vi "TAT-Main.vi"() -> ()   [LabVIEW 2017]
panel:
  in  "Modify SN":bool
  in  "PRINT":bool
  in  "Torque IO Status":bool
  in  "Ass IO Status":bool
  in  "Recipe":bool
  out "error out":errorcluster
  in  "Logout":bool
  in  "Stop":bool
  in  "Create Login":bool
  in  "Reports":bool
  in  "Start":bool
  out "Time":string
  out "Date":string
  in  "Login":bool
  # "RBC ORVM- TRACEABILITY, SCANNING & BARCODE PRINTING"
  # "KAPSE SONS ROBOTICS\n& AUTOMATION"
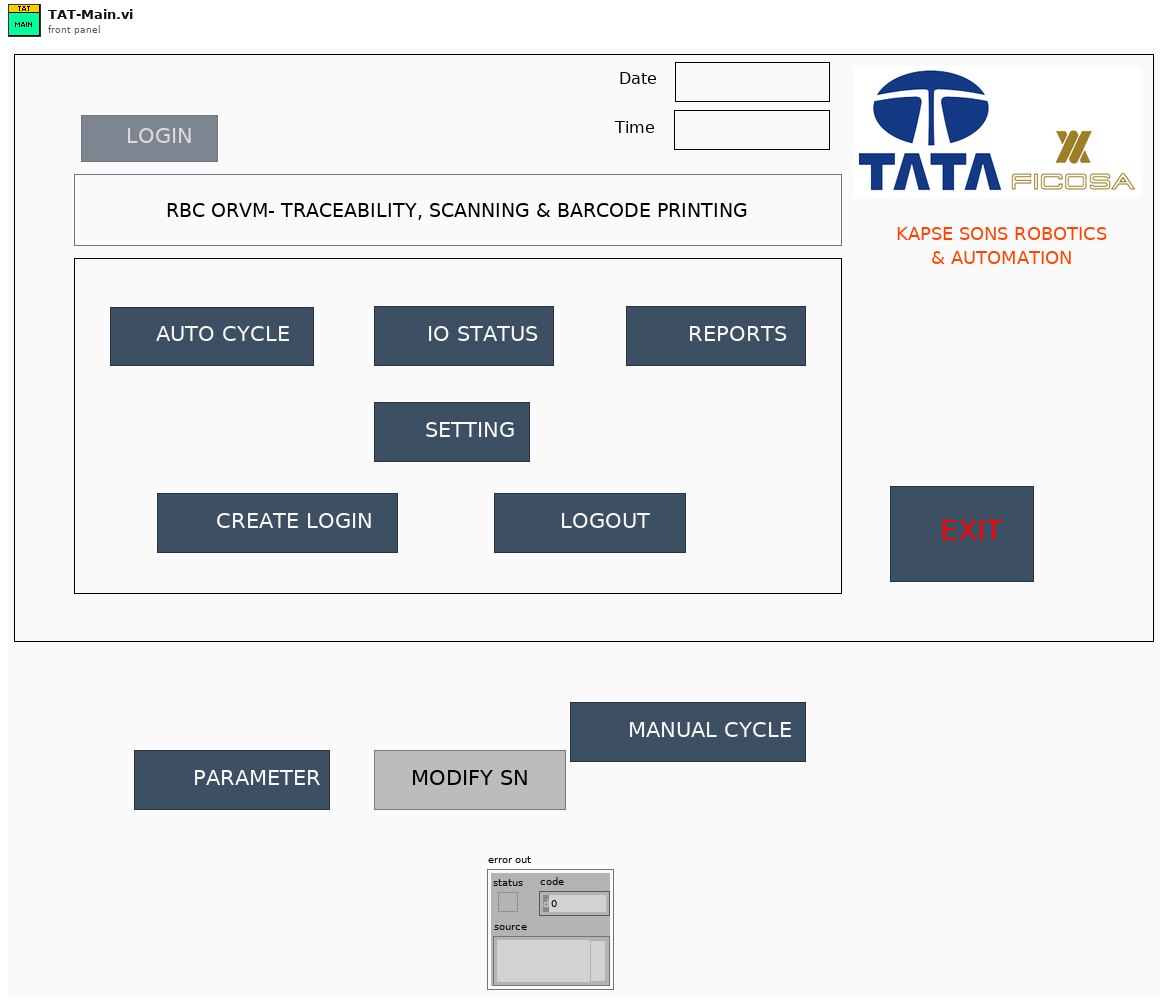
[diagram p1: front panel]
types:
  T1 = enum8{"Enabled", "Disabled", "Disabled and Grayed Out"}
  T2 = enum32{"Invalid", "Standard", "Closed", "Hidden", "Minimized", "Maximized"}
  T3 = enum32{"invalid app kind", "Development System", "Run Time System", "Student Edition", "Embedded LabVIEW", "Evaluation", "Custom"}
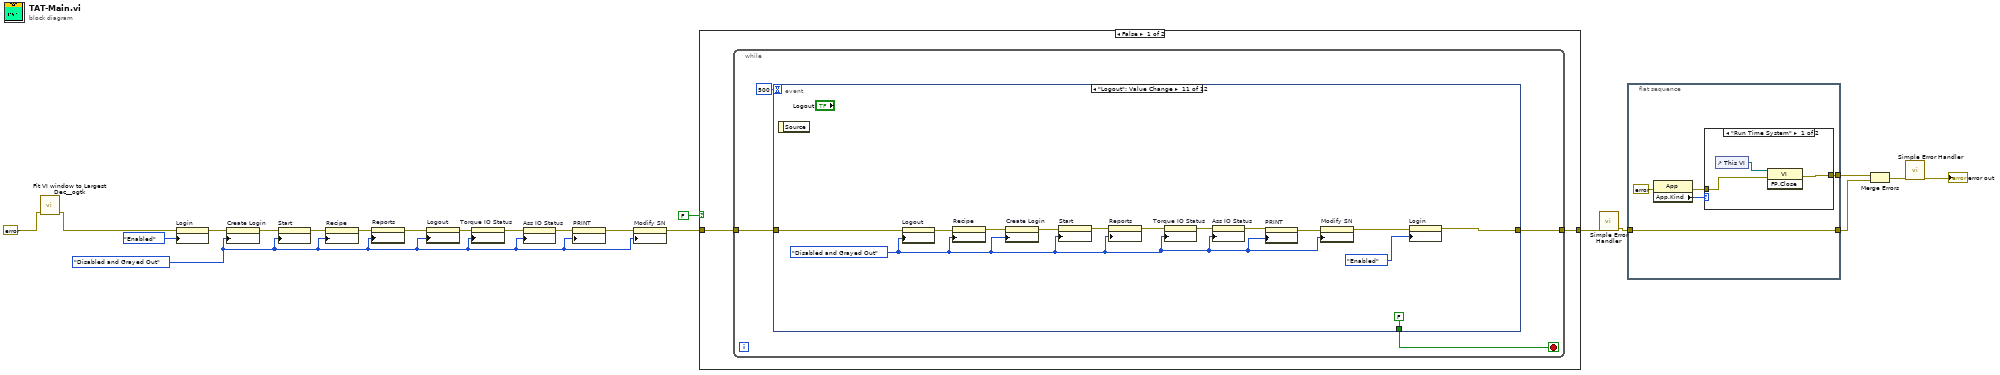
[diagram p0: block diagram]
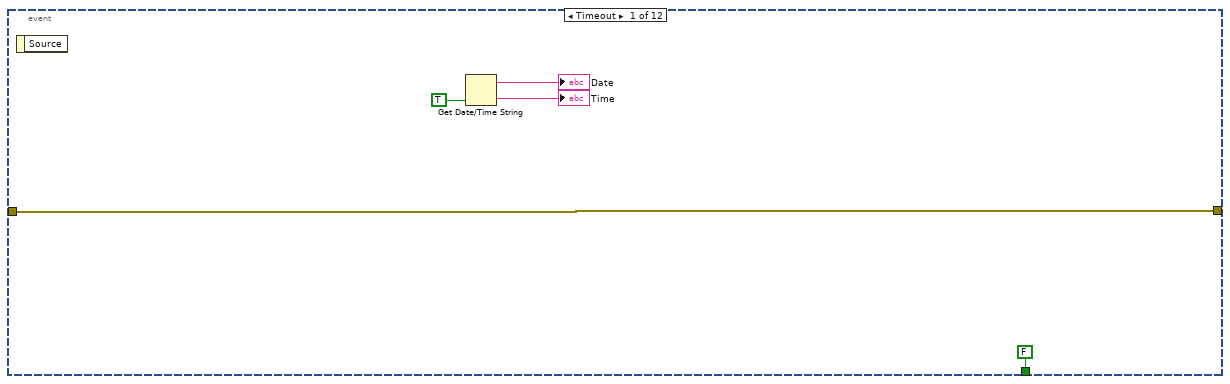
[diagram p3: hidden frame]
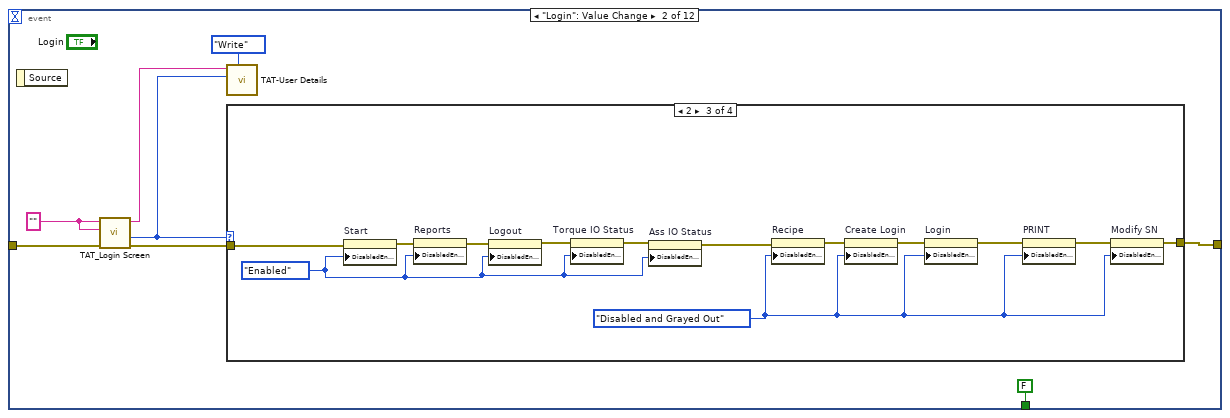
[diagram p4: hidden frame]
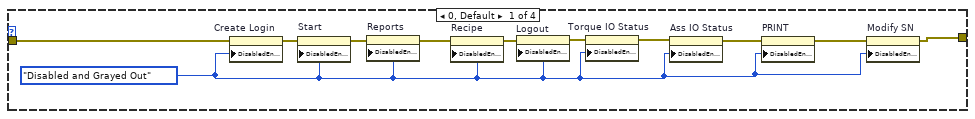
[diagram p5: hidden frame]
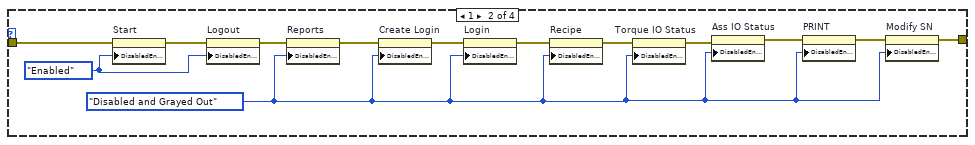
[diagram p6: hidden frame]
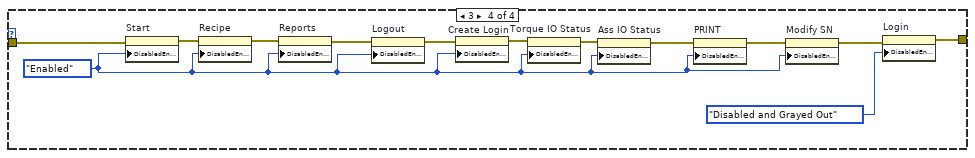
[diagram p7: hidden frame]
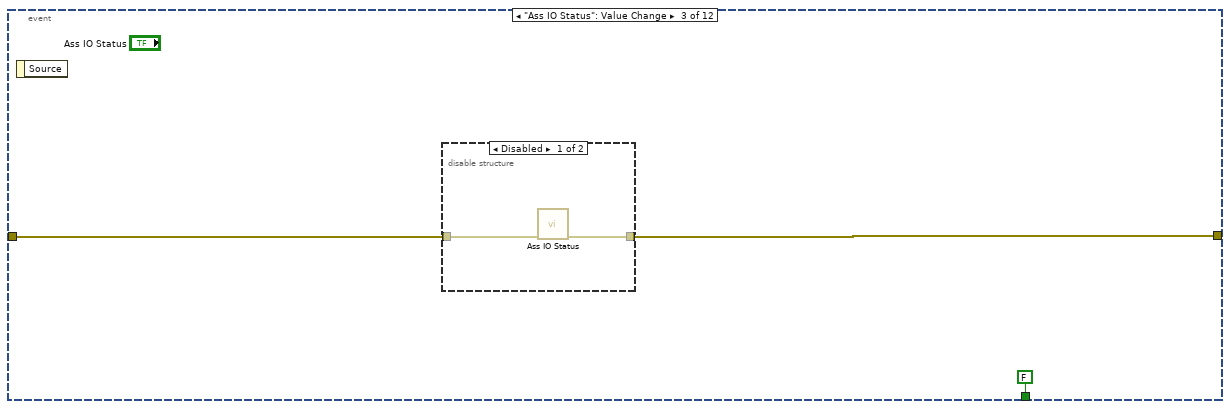
[diagram p8: hidden frame]
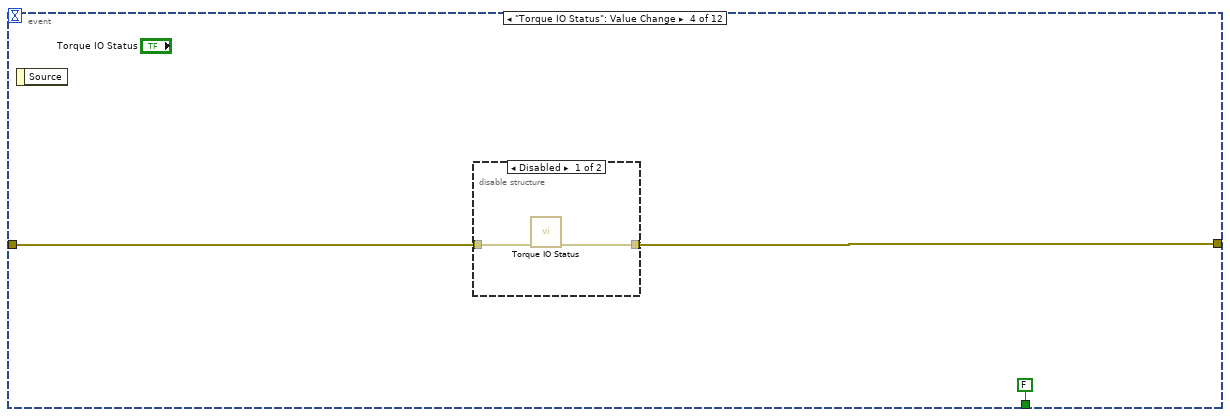
[diagram p10: hidden frame]
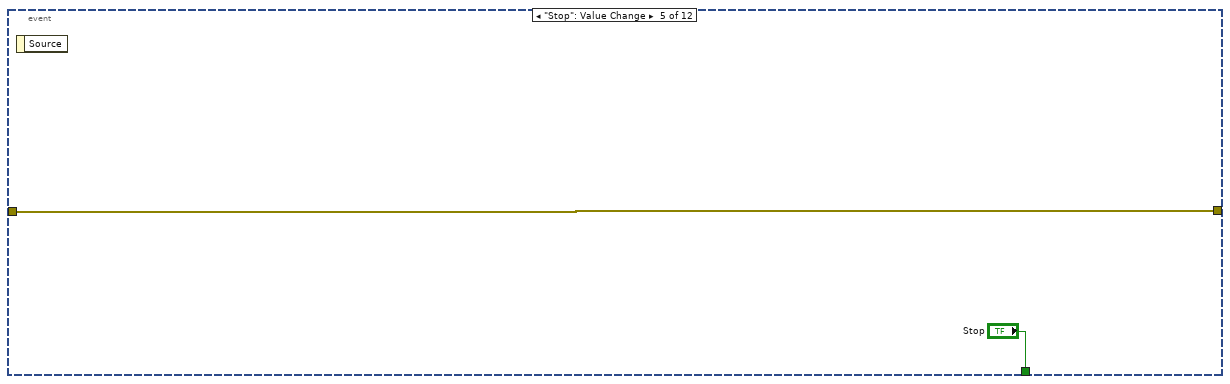
[diagram p12: hidden frame]
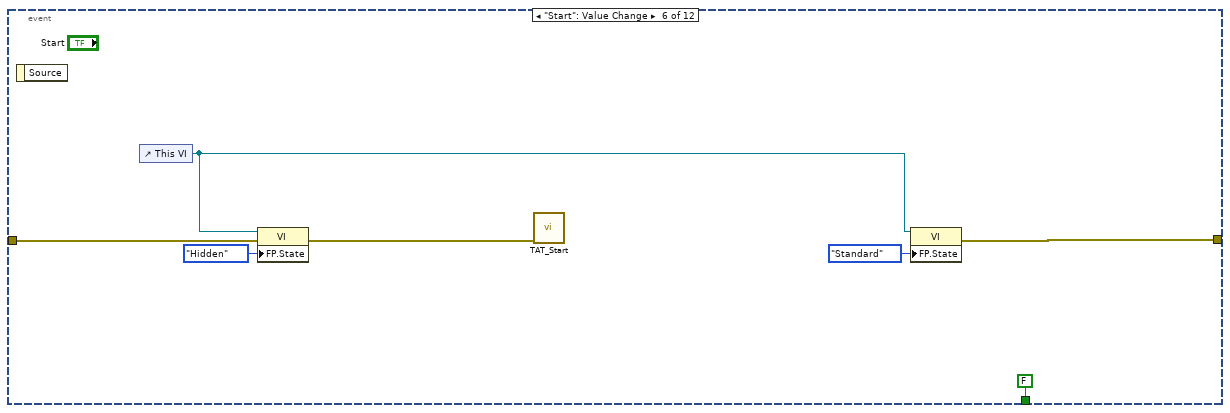
[diagram p13: hidden frame]
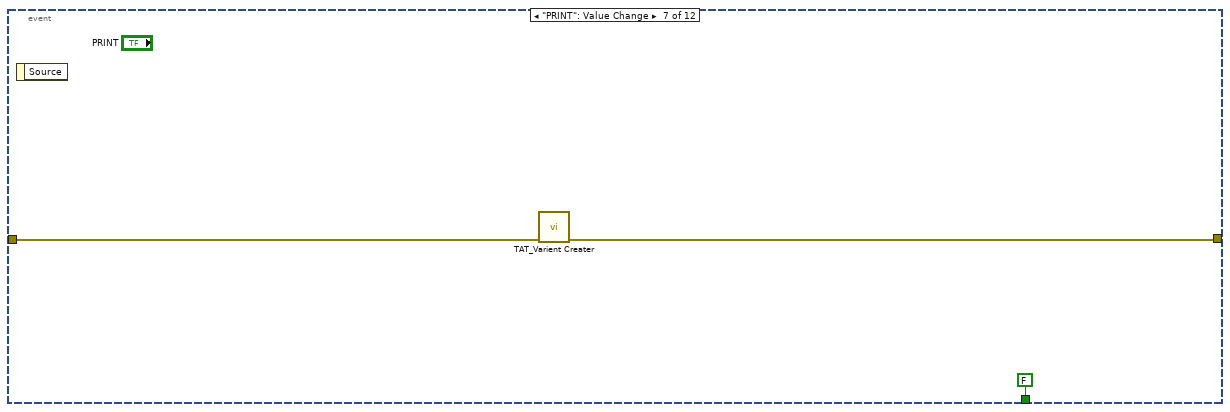
[diagram p14: hidden frame]
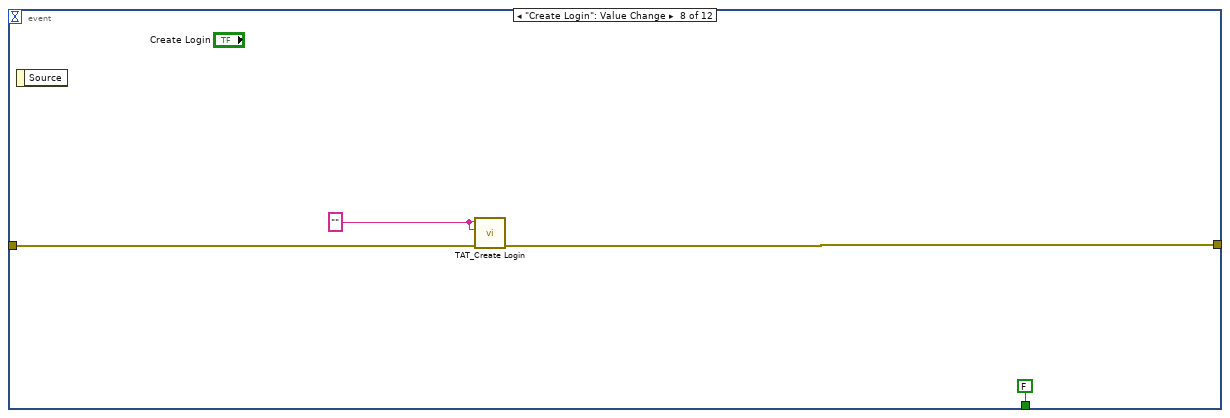
[diagram p15: hidden frame]
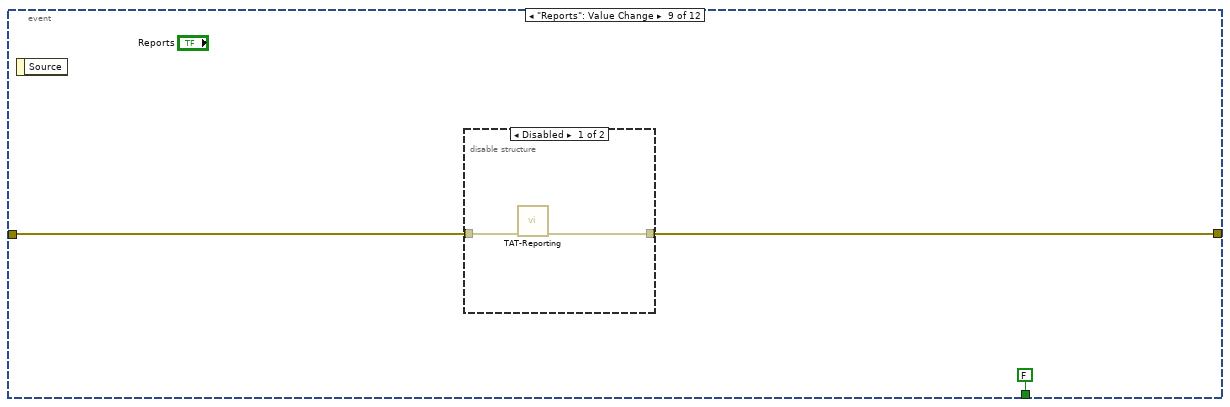
[diagram p16: hidden frame]
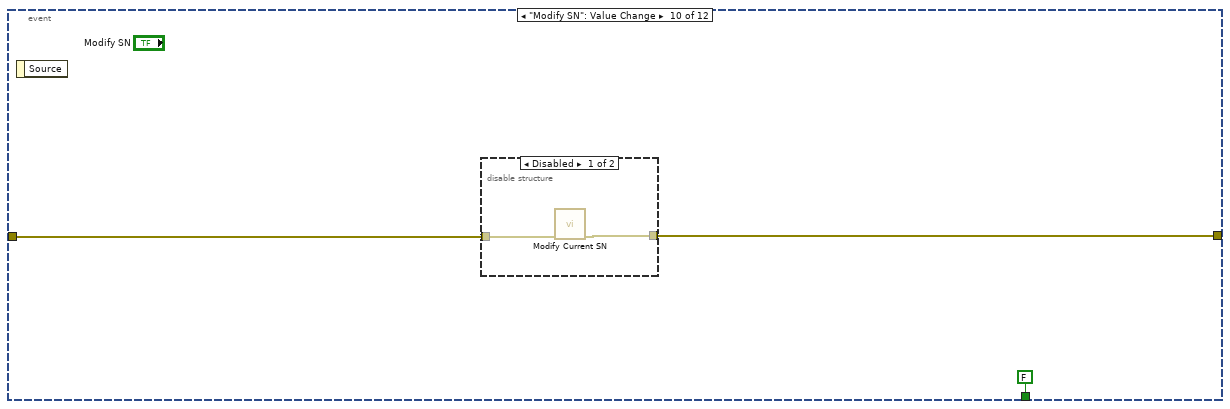
[diagram p18: hidden frame]
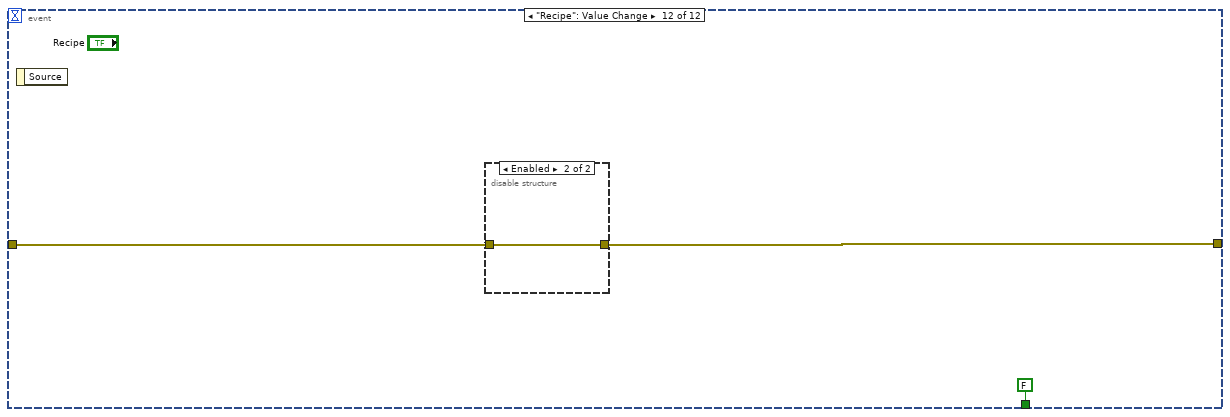
[diagram p20: hidden frame]
diagram:
  w4 = T1."Disabled and Grayed Out" ("Disabled")
  n1 = call <userlib>:"Fit VI window to Largest Dec__ogtk.vi"("error in (no error)"=errorcluster {"status"=FALSE, "code"=0, "source"=""} ("error constant")) -> ("error out"=w1:errorcluster)  [unwired: 5 in, 1 out]
  n2 = property on="Login" class="Bool"(error in=w1, "DisabledEnum"=T1."Enabled" ("Disabled")) -> (error out=w15:errorcluster)  [unwired: 1 in, 1 out]
  n3 = property on="Create Login" class="Bool"(error in=w15, "DisabledEnum"=w4) -> (error out=w20:errorcluster)  [unwired: 1 in, 1 out]
  n4 = property on="Start" class="Bool"(error in=w20, "DisabledEnum"=w4) -> (error out=w11:errorcluster)  [unwired: 1 in, 1 out]
  n5 = property on="Recipe" class="Bool"(error in=w11, "DisabledEnum"=w4) -> (error out=w10:errorcluster)  [unwired: 1 in, 1 out]
  n6 = property on="Reports" class="Bool"(error in=w10, "DisabledEnum"=w4) -> (error out=w13:errorcluster)  [unwired: 1 in, 1 out]
  n7 = property on="Logout" class="Bool"(error in=w13, "DisabledEnum"=w4) -> (error out=w9:errorcluster)  [unwired: 1 in, 1 out]
  n8 = property on="Torque IO Status" class="Bool"(error in=w9, "DisabledEnum"=w4) -> (error out=w8:errorcluster)  [unwired: 1 in, 1 out]
  n9 = property on="Ass IO Status" class="Bool"(error in=w8, "DisabledEnum"=w4) -> (error out=w7:errorcluster)  [unwired: 1 in, 1 out]
  n10 = property on="PRINT" class="Bool"(error in=w7, "DisabledEnum"=w4) -> (error out=w6:errorcluster)  [unwired: 1 in, 1 out]
  n11 = property on="Modify SN" class="Bool"(error in=w6, "DisabledEnum"=w4) -> (error out=w5:errorcluster)  [unwired: 1 in, 1 out]
  n12 = case shown="False" FALSE {
    tunnel: w5 -> [w23 w147]
    tunnel: [w22 w147] -> w21
    frame False {
      n13 = while {
        tunnel: w23 -> [w26]
        tunnel: [w25] -> w22
        stop <- w24 stop-if-true
        n14 = event shown="[10] \"Logout\": Value Change" {
          selector: _ -> [_ _ _ _ _ _ _ _ _ _ _ _]
          dyn-events: _ -> [_ _ _ _ _ _ _ _ _ _ _ _]
          timeout: 500 -> [_ _ _ _ _ _ _ _ _ _ _ _]
          tunnel: w26 -> [w30 w40 w93 w97 w101 w107 w111 w116 w119 w124 w137 w143]
          tunnel: [w30 w38 w92 w96 w101 w104 w110 w115 w118 w123 w138 w142] -> w25
          tunnel: [FALSE ("Stop") FALSE ("Stop") FALSE ("Stop") FALSE ("Stop") "Stop" FALSE ("Stop") FALSE ("Stop") FALSE ("Stop") FALSE ("Stop") FALSE ("Stop") FALSE ("Stop") FALSE ("Stop")] -> w24
          event Timeout {
            n15 = event-data() -> ()  [unwired: 1 in, 1 out]
            n16 = Get Date/Time String(want seconds? (F)=TRUE) -> (date string=→"Date":string, time string=→"Time":string)  [unwired: 2 in]
          }
          event "Login": Value Change {
            w35 = "" ("User Name")
            n17 = event-data() -> ()  [unwired: 1 in, 1 out]
            n18 = call "TAT_Login Screen.vi"("Error In"=w40, "Password"=w35, "User Name"=w35) -> ("error out"=w39:errorcluster, "Level"=w33:i32, "User Name Out"=w36:string)  [unwired: 5 in, 1 out]
            n19 = call "TAT-User Details.vi"("Enum"=enum16{"Read", "Write"}."Write", "Level In"=w33, "User Name In"=w36) -> ()  [unwired: 7 in, 2 out]
            n20 = case shown="2" w33 {
              tunnel: w39 -> [w49 w64 w77 w90]
              tunnel: [w42 w53 w66 w89] -> w38
              frame 0, Default {
                w41 = T1."Disabled and Grayed Out" ("Disabled")
                n21 = property on="Create Login" class="Bool"(error in=w49, "DisabledEnum"=w41) -> (error out=w51:errorcluster)  [unwired: 1 in, 1 out]
                n22 = property on="Start" class="Bool"(error in=w51, "DisabledEnum"=w41) -> (error out=w50:errorcluster)  [unwired: 1 in, 1 out]
                n23 = property on="Reports" class="Bool"(error in=w50, "DisabledEnum"=w41) -> (error out=w48:errorcluster)  [unwired: 1 in, 1 out]
                n24 = property on="Recipe" class="Bool"(error in=w48, "DisabledEnum"=w41) -> (error out=w47:errorcluster)  [unwired: 1 in, 1 out]
                n25 = property on="Logout" class="Bool"(error in=w47, "DisabledEnum"=w41) -> (error out=w46:errorcluster)  [unwired: 1 in, 1 out]
                n26 = property on="Torque IO Status" class="Bool"(error in=w46, "DisabledEnum"=w41) -> (error out=w45:errorcluster)  [unwired: 1 in, 1 out]
                n27 = property on="Ass IO Status" class="Bool"(error in=w45, "DisabledEnum"=w41) -> (error out=w44:errorcluster)  [unwired: 1 in, 1 out]
                n28 = property on="PRINT" class="Bool"(error in=w44, "DisabledEnum"=w41) -> (error out=w43:errorcluster)  [unwired: 1 in, 1 out]
                n29 = property on="Modify SN" class="Bool"(error in=w43, "DisabledEnum"=w41) -> (error out=w42:errorcluster)  [unwired: 1 in, 1 out]
              }
              frame 1 {
                w52 = T1."Disabled and Grayed Out" ("Disabled")
                w60 = T1."Enabled" ("Disabled")
                n30 = property on="Start" class="Bool"(error in=w64, "DisabledEnum"=w60) -> (error out=w59:errorcluster)  [unwired: 1 in, 1 out]
                n31 = property on="Logout" class="Bool"(error in=w59, "DisabledEnum"=w60) -> (error out=w62:errorcluster)  [unwired: 1 in, 1 out]
                n32 = property on="Reports" class="Bool"(error in=w62, "DisabledEnum"=w52) -> (error out=w63:errorcluster)  [unwired: 1 in, 1 out]
                n33 = property on="Create Login" class="Bool"(error in=w63, "DisabledEnum"=w52) -> (error out=w61:errorcluster)  [unwired: 1 in, 1 out]
                n34 = property on="Login" class="Bool"(error in=w61, "DisabledEnum"=w52) -> (error out=w58:errorcluster)  [unwired: 1 in, 1 out]
                n35 = property on="Recipe" class="Bool"(error in=w58, "DisabledEnum"=w52) -> (error out=w56:errorcluster)  [unwired: 1 in, 1 out]
                n36 = property on="Torque IO Status" class="Bool"(error in=w56, "DisabledEnum"=w52) -> (error out=w57:errorcluster)  [unwired: 1 in, 1 out]
                n37 = property on="Ass IO Status" class="Bool"(error in=w57, "DisabledEnum"=w52) -> (error out=w55:errorcluster)  [unwired: 1 in, 1 out]
                n38 = property on="PRINT" class="Bool"(error in=w55, "DisabledEnum"=w52) -> (error out=w54:errorcluster)  [unwired: 1 in, 1 out]
                n39 = property on="Modify SN" class="Bool"(error in=w54, "DisabledEnum"=w52) -> (error out=w53:errorcluster)  [unwired: 1 in, 1 out]
              }
              frame 2 {
                w65 = T1."Disabled and Grayed Out" ("Disabled")
                w69 = T1."Enabled" ("Disabled")
                n40 = property on="Start" class="Bool"(error in=w77, "DisabledEnum"=w69) -> (error out=w74:errorcluster)  [unwired: 1 in, 1 out]
                n41 = property on="Reports" class="Bool"(error in=w74, "DisabledEnum"=w69) -> (error out=w76:errorcluster)  [unwired: 1 in, 1 out]
                n42 = property on="Logout" class="Bool"(error in=w76, "DisabledEnum"=w69) -> (error out=w71:errorcluster)  [unwired: 1 in, 1 out]
                n43 = property on="Torque IO Status" class="Bool"(error in=w71, "DisabledEnum"=w69) -> (error out=w72:errorcluster)  [unwired: 1 in, 1 out]
                n44 = property on="Ass IO Status" class="Bool"(error in=w72, "DisabledEnum"=w69) -> (error out=w70:errorcluster)  [unwired: 1 in, 1 out]
                n45 = property on="Recipe" class="Bool"(error in=w70, "DisabledEnum"=w65) -> (error out=w73:errorcluster)  [unwired: 1 in, 1 out]
                n46 = property on="Create Login" class="Bool"(error in=w73, "DisabledEnum"=w65) -> (error out=w75:errorcluster)  [unwired: 1 in, 1 out]
                n47 = property on="Login" class="Bool"(error in=w75, "DisabledEnum"=w65) -> (error out=w68:errorcluster)  [unwired: 1 in, 1 out]
                n48 = property on="PRINT" class="Bool"(error in=w68, "DisabledEnum"=w65) -> (error out=w67:errorcluster)  [unwired: 1 in, 1 out]
                n49 = property on="Modify SN" class="Bool"(error in=w67, "DisabledEnum"=w65) -> (error out=w66:errorcluster)  [unwired: 1 in, 1 out]
              }
              frame 3 {
                w78 = T1."Enabled" ("Disabled")
                n50 = property on="Start" class="Bool"(error in=w90, "DisabledEnum"=w78) -> (error out=w85:errorcluster)  [unwired: 1 in, 1 out]
                n51 = property on="Recipe" class="Bool"(error in=w85, "DisabledEnum"=w78) -> (error out=w84:errorcluster)  [unwired: 1 in, 1 out]
                n52 = property on="Reports" class="Bool"(error in=w84, "DisabledEnum"=w78) -> (error out=w87:errorcluster)  [unwired: 1 in, 1 out]
                n53 = property on="Logout" class="Bool"(error in=w87, "DisabledEnum"=w78) -> (error out=w86:errorcluster)  [unwired: 1 in, 1 out]
                n54 = property on="Create Login" class="Bool"(error in=w86, "DisabledEnum"=w78) -> (error out=w83:errorcluster)  [unwired: 1 in, 1 out]
                n55 = property on="Torque IO Status" class="Bool"(error in=w83, "DisabledEnum"=w78) -> (error out=w82:errorcluster)  [unwired: 1 in, 1 out]
                n56 = property on="Ass IO Status" class="Bool"(error in=w82, "DisabledEnum"=w78) -> (error out=w81:errorcluster)  [unwired: 1 in, 1 out]
                n57 = property on="PRINT" class="Bool"(error in=w81, "DisabledEnum"=w78) -> (error out=w80:errorcluster)  [unwired: 1 in, 1 out]
                n58 = property on="Modify SN" class="Bool"(error in=w80, "DisabledEnum"=w78) -> (error out=w79:errorcluster)  [unwired: 1 in, 1 out]
                n59 = property on="Login" class="Bool"(error in=w79, "DisabledEnum"=T1."Disabled and Grayed Out" ("Disabled")) -> (error out=w89:errorcluster)  [unwired: 1 in, 1 out]
              }
            }
          }
          event "Ass IO Status": Value Change {
            n60 = event-data() -> ()  [unwired: 1 in, 1 out]
            n61 = disable-structure shown="Disabled" {
              disable-tunnel: w93 -> [w95 _]
              disable-tunnel: [w94 _] -> w92
              frame Disabled {
                n62 = call "Ass IO Status.vi"("error in (no error)"=w95) -> ("error out"=w94:errorcluster)  [unwired: 10 in]
              }
              frame Enabled {
              }
            }
          }
          event "Torque IO Status": Value Change {
            n63 = event-data() -> ()  [unwired: 1 in, 1 out]
            n64 = disable-structure shown="Disabled" {
              disable-tunnel: w97 -> [w100 _]
              disable-tunnel: [w99 _] -> w96
              frame Disabled {
                n65 = call "Torque IO Status.vi"("error in (no error)"=w100) -> ("error out"=w99:errorcluster)  [unwired: 10 in]
              }
              frame Enabled {
              }
            }
          }
          event "Stop": Value Change {
            n66 = event-data() -> ()  [unwired: 1 in, 1 out]
          }
          event "Start": Value Change {
            n67 = event-data() -> ()  [unwired: 1 in, 1 out]
            n68 = control-ref of="This VI"() -> (w105:refnum<vi>)
            n69 = property class="VI"(reference=w105, error in=w107, "FP.State"=T2."Hidden" ("Front Panel Window:State")) -> (error out=w103:errorcluster)  [unwired: 1 out]
            n70 = call "TAT_Start.vi"("error In"=w103) -> ()  [unwired: 11 in]
            n71 = property class="VI"(reference=w105, "FP.State"=T2."Standard" ("Front Panel Window:State")) -> (error out=w104:errorcluster)  [unwired: 1 in, 1 out]
          }
          event "PRINT": Value Change {
            n72 = event-data() -> ()  [unwired: 1 in, 1 out]
            n73 = call "TAT_Varient Creater.vi"("error in (no error)"=w111) -> ("error out"=w110:errorcluster)  [unwired: 10 in]
          }
          event "Create Login": Value Change {
            w114 = "" ("User Name")
            n74 = event-data() -> ()  [unwired: 1 in, 1 out]
            n75 = call "TAT_Create Login.vi"("Error In"=w116, "Password"=w114, "User Name"=w114) -> ("error out"=w115:errorcluster)  [unwired: 6 in]
          }
          event "Reports": Value Change {
            n76 = event-data() -> ()  [unwired: 1 in, 1 out]
            n77 = disable-structure shown="Disabled" {
              disable-tunnel: w119 -> [w121 _]
              disable-tunnel: [w120 _] -> w118
              frame Disabled {
                n78 = call "TAT-Reporting.vi"("error in (no error)"=w121) -> ("error out"=w120:errorcluster)  [unwired: 10 in]
              }
              frame Enabled {
              }
            }
          }
          event "Modify SN": Value Change {
            n79 = event-data() -> ()  [unwired: 1 in, 1 out]
            n80 = disable-structure shown="Disabled" {
              disable-tunnel: w124 -> [w126 _]
              disable-tunnel: [w125 _] -> w123
              frame Disabled {
                n81 = call "Modify Current SN.vi"("error in (no error)"=w126) -> ("error out"=w125:errorcluster)  [unwired: 10 in]
              }
              frame Enabled {
              }
            }
          }
          event "Logout": Value Change {
            w127 = T1."Disabled and Grayed Out" ("Disabled")
            n82 = event-data() -> ()  [unwired: 1 in, 1 out]
            n83 = property on="Logout" class="Bool"(error in=w137, "DisabledEnum"=w127) -> (error out=w135:errorcluster)  [unwired: 1 in, 1 out]
            n84 = property on="Recipe" class="Bool"(error in=w135, "DisabledEnum"=w127) -> (error out=w134:errorcluster)  [unwired: 1 in, 1 out]
            n85 = property on="Create Login" class="Bool"(error in=w134, "DisabledEnum"=w127) -> (error out=w140:errorcluster)  [unwired: 1 in, 1 out]
            n86 = property on="Start" class="Bool"(error in=w140, "DisabledEnum"=w127) -> (error out=w139:errorcluster)  [unwired: 1 in, 1 out]
            n87 = property on="Reports" class="Bool"(error in=w139, "DisabledEnum"=w127) -> (error out=w132:errorcluster)  [unwired: 1 in, 1 out]
            n88 = property on="Torque IO Status" class="Bool"(error in=w132, "DisabledEnum"=w127) -> (error out=w133:errorcluster)  [unwired: 1 in, 1 out]
            n89 = property on="Ass IO Status" class="Bool"(error in=w133, "DisabledEnum"=w127) -> (error out=w130:errorcluster)  [unwired: 1 in, 1 out]
            n90 = property on="PRINT" class="Bool"(error in=w130, "DisabledEnum"=w127) -> (error out=w129:errorcluster)  [unwired: 1 in, 1 out]
            n91 = property on="Modify SN" class="Bool"(error in=w129, "DisabledEnum"=w127) -> (error out=w128:errorcluster)  [unwired: 1 in, 1 out]
            n92 = property on="Login" class="Bool"(error in=w128, "DisabledEnum"=T1."Enabled" ("Disabled")) -> (error out=w138:errorcluster)  [unwired: 1 in, 1 out]
          }
          event "Recipe": Value Change {
            n93 = event-data() -> ()  [unwired: 1 in, 1 out]
            n94 = disable-structure shown="Enabled" {
              disable-tunnel: w143 -> [w145 w146]
              disable-tunnel: [w144 w146] -> w142
              frame Disabled {
                n95 = call "TAT-Create Reciepe.vi"("Error In"=w145) -> ("error out"=w144:errorcluster)  [unwired: 10 in]
              }
              frame Enabled {
              }
            }
          }
        }
      }
    }
    frame True {
    }
  }
  n96 = call <vilib>:"Simple Error Handler.vi"("error in (no error)"=w21) -> ("error out"=w16:errorcluster)  [unwired: 4 in, 4 out]
  n97 = flat-sequence {
    tunnel: [w149] -> w19
    tunnel: [w148] -> w17
    tunnel: w16 -> [w148]
    frame #0 {
      n98 = property class="App"(error in=errorcluster {"status"=FALSE, "code"=0, "source"=""} ("error in (no error)")) -> (error out=w151:errorcluster, "App.Kind"=w152:T3)  [unwired: 1 in, 1 out]
      n99 = case shown="\"Run Time System\"" w152 {
        tunnel: w151 -> [w154 w156]
        tunnel: [w153 w156] -> w149
        frame "Run Time System" {
          n100 = control-ref of="This VI"() -> (w155:refnum<vi>)
          n101 = invoke class="VI" method="FP.Close"(reference=w155, error in=w154) -> (error out=w153:errorcluster)  [unwired: 1 in, 2 out]
        }
        frame "Development System", Default {
        }
      }
    }
  }
  n102 = Merge Errors(w19, w17) -> (w18:errorcluster)
  n103 = call <vilib>:"Simple Error Handler.vi"("error in (no error)"=w18) -> ("error out"=→"error out":errorcluster)  [unwired: 4 in, 4 out]
